vi "Populate Variables in CMD.vi"(5 "Variant":variant, 6 "Error in":errorcluster caption="Error in (no error)", 9 "String might with variables":string) -> (0 "Error out":errorcluster, 3 "String out":string, 4 "Variant Out":variant)   [LabVIEW 2020, in "CSMScript-Engine(Lite).lvlib"]
uses:
  CSMScript-Engine(Lite).lvlib
  <userlib>/_NEVSTOP/Communicable State Machine(CSM)/_Shared/CSM Shared.lvlib
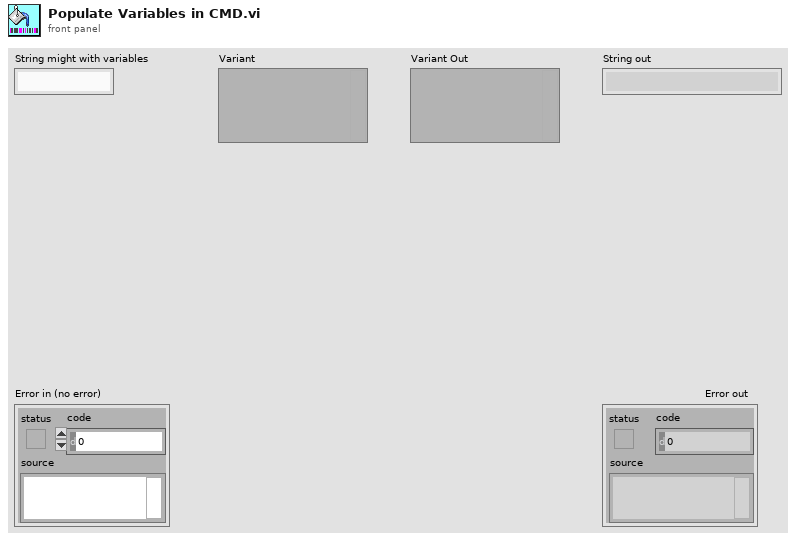
[diagram p1: front panel]
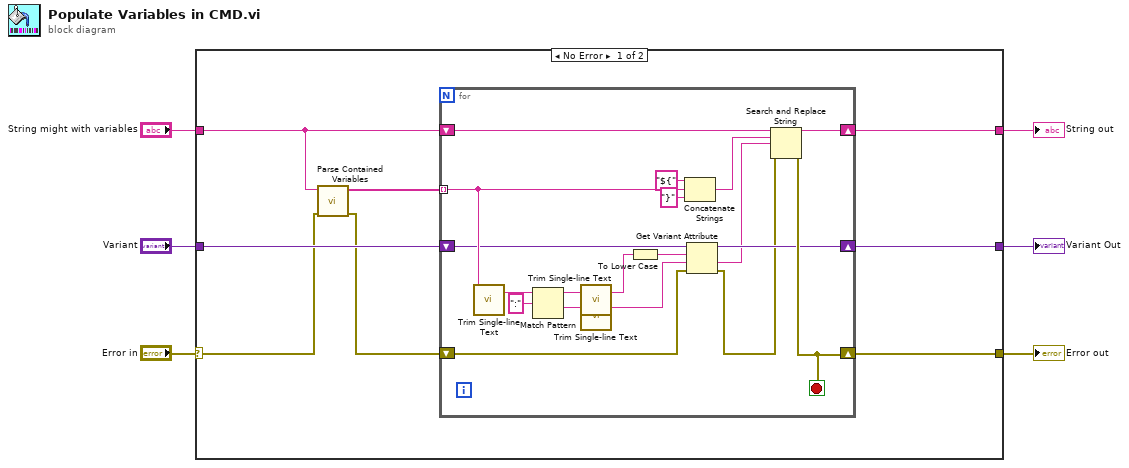
[diagram p0: block diagram]
diagram:
  n1 = case shown="No Error" "Error in" {
    selector: "Error in" -> [w8 w36]
    tunnel: [w14 w35] -> w6
    tunnel: "String might with variables" -> [w13 w35]
    tunnel: [w12 w36] -> w3
    tunnel: "Variant" -> [w11 w34]
    tunnel: [w10 w34] -> w1
    frame No Error {
      n2 = call <userlib>:"Parse Contained Variables.vi"("Error in"=w8, "String"=w13) -> ("Error out"=w7:errorcluster, "Contained Variables"=w9:string[])  [unwired: 8 in]
      n3 = for {
        tunnel: w9 -> [w31] mode=indexing
        shift-right: [w32] -> w14
        shift-left: w13 -> [w33]
        shift-right: [w30] -> w12
        shift-left: w7 -> [w29]
        shift-right: [w20] -> w10
        shift-left: w11 -> [w28]
        stop <- w30 stop-if-true
        n4 = call <userlib>:"Trim Single-line Text.vi"("single-line text"=w31) -> ("trimed text"=w23:string)  [unwired: 2 in]
        n5 = Match Pattern(string=w23, regular expression=":") -> (before substring=w26:string, after substring=w25:string)  [unwired: 1 in, 2 out]
        n6 = call <userlib>:"Trim Single-line Text.vi"("single-line text"=w26) -> ("trimed text"=w22:string)  [unwired: 2 in]
        n7 = call <userlib>:"Trim Single-line Text.vi"("single-line text"=w25) -> ("trimed text"=w24:string)  [unwired: 2 in]
        n8 = To Lower Case(string=w22) -> (all lower case string=w21:string)
        n9 = Concatenate Strings("${" ("regular expression"), w31, "}" ("regular expression")) -> (w15:string)
        n10 = Get Variant Attribute(Variant=w28, name=w21, default value (empty Variant)=w24, error in=w29) -> (duplicate Variant=w20:variant, value=w19:string, error out=w18:errorcluster)  [unwired: 1 out]
        n11 = Search and Replace String(input string=w33, search string=w15, replace string=w19, error in=w18) -> (result string=w32:string, error out=w30:errorcluster)  [unwired: 4 in, 2 out]
      }
    }
    frame Error {
    }
  }
  "String out" <- w6
  "Error out" <- w3
  "Variant Out" <- w1
